vi "HEWH Read Resistance Example.vi"() -> ()   [LabVIEW 2020]
uses:
  Agilent 34970.lvlib
panel:
  out "error out":errorcluster
  out "Temperature (F)":dbl
  in  "stop":bool
  out "Thermistor Reading (kOhms)":dbl
  in  "VISA Refnum in":refnum<visa-resource-name>
  in  "Error In":errorcluster
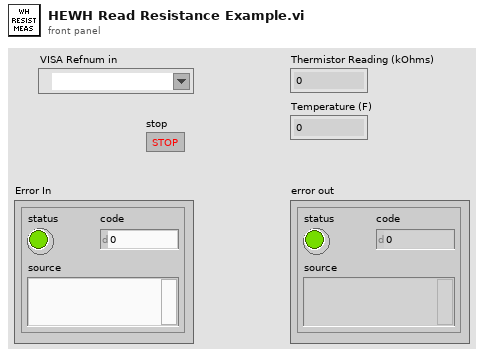
[diagram p1: front panel]
types:
  T1 = enum16{"100 Ohm", "1 kOhm", "10 kOhm", "100 kOhm", "1 MOhm", "10 MOhm", "100 MOhm", "Minimum", "Maximum"}
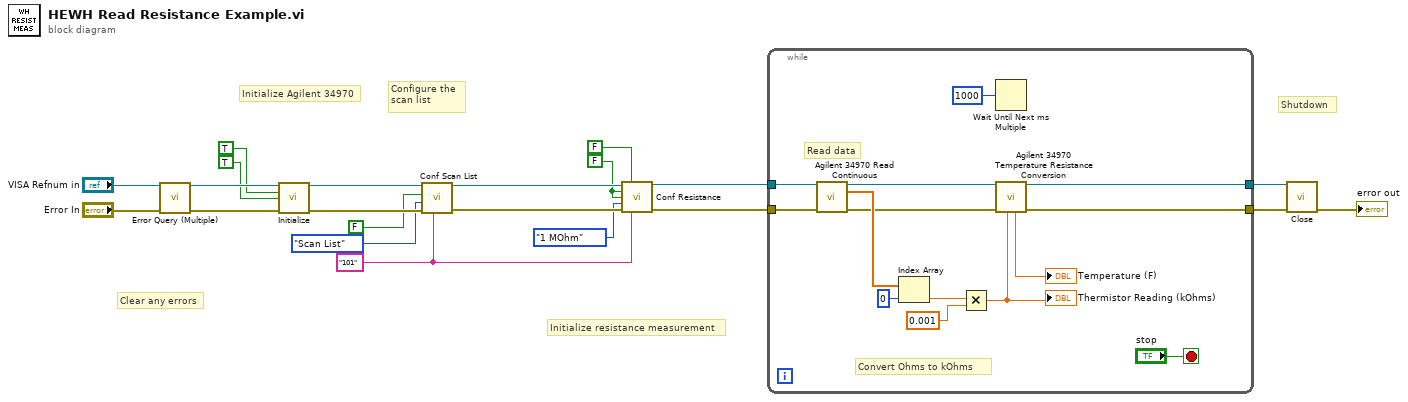
[diagram p0: block diagram]
diagram:
  w5 = FALSE ("4 Wire/2 Wire (F:2)")
  w9 = "101" ("Channel List (empty)")
  # "Initialize resistance measurement"
  # "Configure the\nscan list"
  # "Shutdown"
  # "Clear any errors"
  # "Initialize Agilent 34970"
  n1 = call "Error Query (Multiple).vi"("VISA Resource Name"="VISA Refnum in", "error in (no error)"="Error In") -> ("VISA Resource Name Out"=w20:refnum<visa-resource-name>, "error out"=w19:errorcluster)  [unwired: 10 in, 2 out]
  n2 = call "Initialize.vi"("VISA Resource Name"=w20, "ID Query (T: Check)"=TRUE, "Reset (T: Reset)"=TRUE, "error in (no error)"=w19) -> ("VISA Resource Name Out"=w13:refnum<visa-resource-name>, "error out"=w12:errorcluster)  [unwired: 10 in]
  n3 = call "Conf Scan List.vi"("Scan List (empty)"=w9, "error in (no error)"=w12, "Check Parameter (0:Scan List)"=enum16{"Scan List", "Scan Size"}."Scan List", "Set/Check (F:Set)"=FALSE, "VISA Resource Name"=w13) -> ("error out"=w11:errorcluster, "VISA Resource Name Out"=w10:refnum<visa-resource-name>)  [unwired: 4 in, 1 out]
  n4 = call "Conf Resistance.vi"("VISA Resource Name"=w10, "Check/Set (F:Set)"=FALSE, "4 Wire/2 Wire (F:2)"=w5, "Autorange? (F:OFF)"=w5, "Range (8:Maximum)"=T1."1 MOhm", "error in (no error)"=w11, "Channel List (empty)"=w9) -> ("VISA Resource Name Out"=w3:refnum<visa-resource-name>, "error out"=w2:errorcluster)  [unwired: 6 in, 1 out]
  n5 = while {
    tunnel: w3 -> [w33]
    tunnel: [w34] -> w15
    tunnel: w2 -> [w32]
    tunnel: [w24] -> w14
    stop <- "stop" stop-if-true
    # "Convert Ohms to kOhms"
    # "Read data"
    n6 = call "Agilent 34970 Read Continuous.vi"("VISA Resource Name"=w33, "error in (no error)"=w32) -> ("VISA resource name out"=w34:refnum<visa-resource-name>, "Output Array"=w31:dbl[], "error out"=w25:errorcluster)  [unwired: 10 in, 1 out]
    n7 = Index Array(array=w31, index=0) -> (element=w29:dbl)
    n8 = Multiply(x=w29, y=0.001) -> (x*y=w23:dbl)
    "Thermistor Reading (kOhms)" <- w23
    n9 = Wait Until Next ms Multiple(millisecond multiple=u32 1000) -> ()  [unwired: 1 out]
    n10 = call "Agilent 34970 Temperature Resistance Conversion.vi"("Resistance Value"=w23, "error in (no error)"=w25) -> ("error out"=w24:errorcluster, "Temperature (F)"=→"Temperature (F)":dbl)  [unwired: 8 in]
  }
  n11 = call "Close.vi"("VISA Resource Name"=w15, "error in (no error)"=w14) -> ("error out"=→"error out":errorcluster)  [unwired: 13 in]
